vi "Search Sysdef for Targets.vi"(8 "error in (no error)":errorcluster, 11 "NIVS.System Definition Root":refnum<k24>) -> (0 "error out":errorcluster, 1 "Target Names":string[](array[string]), 3 "NIVS.System Defintion Root Out":refnum<k24>, 5 "Windows?":bool[](array[boolean]), 7 "Target Nodes":refnum<k24>[](array[refnum]))   [LabVIEW 2011]
uses:
  NationalInstruments.VeriStand.SystemStorage
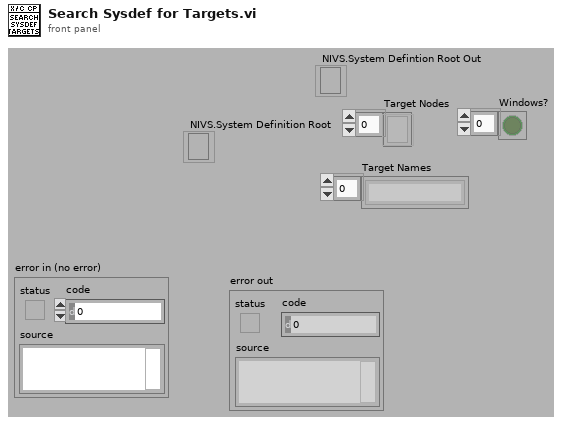
[diagram p1: front panel]
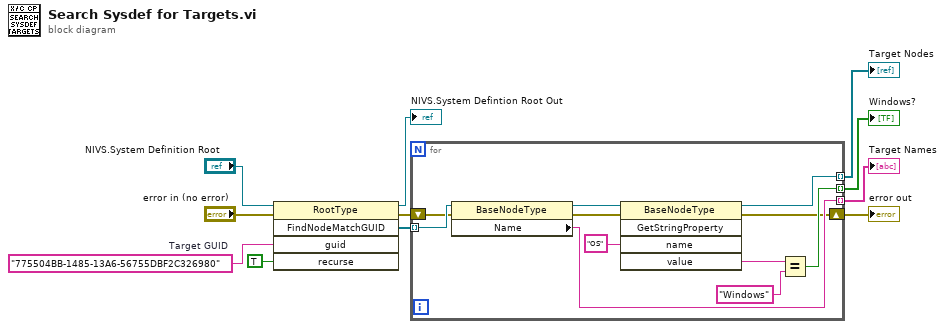
[diagram p0: block diagram]
diagram:
  w5 = "775504BB-1485-13A6-56755DBF2C326980"  # Target GUID
  n1 = invoke class="RootType" method="FindNodeMatchGUID"(reference="NIVS.System Definition Root", error in="error in (no error)", "guid"=w5, "recurse"=TRUE) -> (reference out=→"NIVS.System Defintion Root Out":refnum<k24>, error out=w3:errorcluster, "FindNodeMatchGUID"=w4:refnum<k24>[])  [unwired: 1 in, 2 out]
  n2 = for {
    tunnel: w4 -> [w22] mode=indexing
    shift-right: [w12] -> w6
    shift-left: w3 -> [w20]
    tunnel: [w17] -> w8 mode=indexing
    tunnel: [w21] -> w7 mode=indexing
    tunnel: [w13] -> w1 mode=indexing
    n3 = property class="BaseNodeType"(reference=w22, error in=w20) -> (reference out=w18:refnum<k24>, error out=w19:errorcluster, "Name"=w21:string)
    n4 = invoke class="BaseNodeType" method="GetStringProperty"(reference=w18, error in=w19, "name"="OS") -> (reference out=w17:refnum<k24>, error out=w12:errorcluster, "value"=w15:string)  [unwired: 2 in, 2 out]
    n5 = Equal?(x=w15, y="Windows") -> (x = y?=w13:bool)
  }
  "error out" <- w6
  "Target Nodes" <- w8
  "Target Names" <- w7
  "Windows?" <- w1
